vi "Channel.Config to Runtime.vi"(8 "error in (no error)":errorcluster, 9 "access":T1, 10 "Channel Configuration":refnum<class "Configuration.Channel.lvclass">, 11 "Device Ref in":T2=18446744073709551615 format="%.0x") -> (0 "error out":errorcluster, 2 "Channel Runtime":refnum<class "Runtime.Channel.lvclass">, 3 "Device Ref out":T2=18446744073709551615 format="%.0x")   [LabVIEW 2016, in "Data Sharing Framework.Runtime.lvlib"]
uses:
  Data Sharing Framework.Runtime.lvlib
  Classes/Runtime/Channel/Runtime.Channel.lvclass
  Classes/Configuration.Channel/Configuration.Channel.lvclass
  <vilib>/NI Veristand/Custom Device API/Custom Device Item Ref.ctl
  <vilib>/NI Veristand/Custom Device API/Data Access Type.ctl
  Classes/Configuration.Channel/Configuration.Channel.lvclass/Configuration.Channel.ctl
  Classes/Runtime/Channel/Runtime.Channel.lvclass/Runtime.Channel.ctl
  <vilib>/NI Veristand/VeriStand Data/Data Channels/Channels.Inline.Reference Error Handler.vi
  <vilib>/NI Veristand/Custom Device API/Global Data Refs.vi
  <vilib>/NI VeriStand/Custom Device API/Custom Device API.lvlib
  <vilib>/NI Veristand/VeriStand Data/VeriStand Data.lvlib
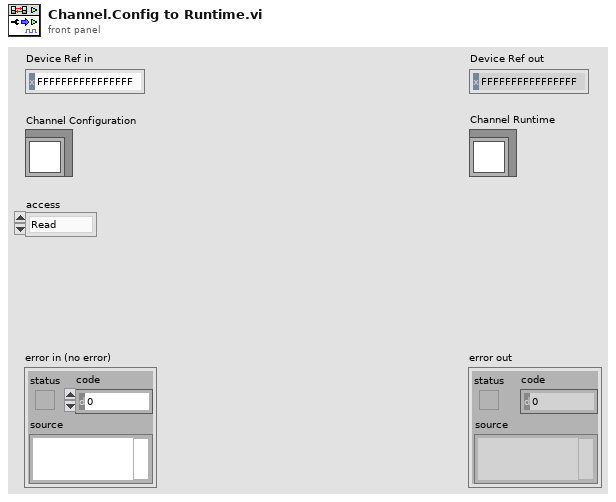
[diagram p1: front panel]
types:
  T1 = typedef "Custom Device API.lvlib/Data Access Type.ctl" = enum16{"Read", "Write"}
  T2 = typedef "Custom Device API.lvlib/Custom Device Item Ref.ctl" = u64
  T3 = typedef "Data Sharing Framework.Configuration.lvlib/Configuration.Channel.lvclass/Channel Configuration.ctl" = cluster{"data type":T4, "offset":u64}
  T4 = typedef "VeriStand Data.lvlib/Typedefs.Data Types.ctl" = enum16{"Boolean", "Single", "Double", "I8", "I16", "I32", "I64", "U8", "U16", "U32", "U64"}
  T5 = typedef "Custom Device API.lvlib/Data Reference.ctl" = i32
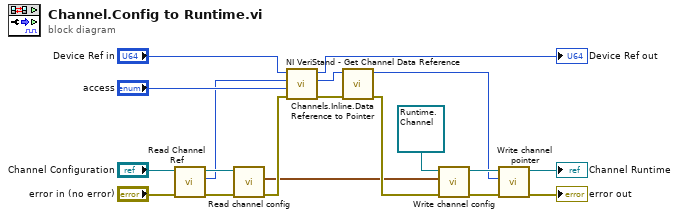
[diagram p0: block diagram]
diagram:
  n1 = call "Read Channel Ref.vi"("error in (no error)"="error in (no error)", "Configuration.Channel in"="Channel Configuration") -> ("error out"=w8:errorcluster, "Channel Ref"=w7:T2, "Configuration.Channel out"=w9:refnum<class "Configuration.Channel.lvclass">)  [unwired: 7 in]
  n2 = call "Read channel config.vi"("error in (no error)"=w8, "Configuration.Channel in"=w9) -> ("error out"=w3:errorcluster, "channel config"=w1:T3)  [unwired: 7 in, 1 out]
  n3 = call <vilib>:"NI VeriStand - Get Channel Data Reference.vi"("error in (no error)"=w3, "Access"="access", "Channel Ref in"=w7, "Device Ref in"="Device Ref in") -> ("error out"=w16:errorcluster, "Channel Data Reference"=w15:T5, "Device Ref out"=→"Device Ref out":T2)  [unwired: 5 in]
  n4 = call <vilib>:"Channels.Inline.Data Reference to Pointer.vi"("error in (no error)"=w16, "Data Reference in"=w15) -> ("error out"=w2:errorcluster, "Channel Pointer"=w4:u64)  [unwired: 8 in]
  n5 = call "Write channel config.vi"("error in (no error)"=w2, "channel config"=w1, "Runtime.Channel in"=refnum<class "Runtime.Channel.lvclass"> refnum ("Channel Runtime")) -> ("error out"=w5:errorcluster, "Runtime.Channel out"=w6:refnum<class "Runtime.Channel.lvclass">)  [unwired: 7 in]
  n6 = call "Write channel pointer.vi"("error in (no error)"=w5, "channel pointer"=w4, "Runtime.Channel in"=w6) -> ("error out"=→"error out":errorcluster, "Runtime.Channel out"=→"Channel Runtime":refnum<class "Runtime.Channel.lvclass">)  [unwired: 7 in]
